vi "Apply Target Pattern.vi"(10 "Mixed Mode Status":T3={"LBCB Target"=[], "MixedModeStates"=enum."Idle", "LBCB Convergence"=[], "LBCB Measurements"=[]}, 11 "Target Pattern":T8) -> (2 "Targets":T1[](array[typedef]))   [LabVIEW 2009]
uses:
  Target Pattern.ctl
  MixedMode/Messages/Target.ctl
  Data Access Objects/Metadata/LBCB Number.ctl
  MixedMode/Messages/Mixed Mode Status.ctl
  MixedMode/Target Data.ctl
  MixedMode/Mixed Mode States.ctl
  MixedMode/Mixed Mode Covergance Status.ctl
  MixedMode/Mixed Mode Cartesian Data.ctl
panel:
  in  "Moments":T1[](array[typedef])=[{"LBCB Number"=enum."LBCB1", "DOF Vectors"=enum."Mx", "Amount"=0.0}, {"LBCB Number"=enum."LBCB1", "DOF Vectors"=enum."My", "Amount"=0.0}, {"LBCB Number"=enum."LBCB1", "DOF Vectors"=enum."Mz", "Amount"=0.0}, {"LBCB Number"=enum."LBCB2", "DOF Vectors"=enum."Mx", "Amount"=0.0}, {"LBCB Number"=enum."LBCB2", "DOF Vectors"=enum."My", "Amount"=0.0}, {"LBCB Number"=enum."LBCB2", "DOF Vectors"=enum."Mz", "Amount"=0.0}]
  in  "Forces":T1[](array[typedef])=[{"LBCB Number"=enum."LBCB1", "DOF Vectors"=enum."Fx", "Amount"=0.0}, {"LBCB Number"=enum."LBCB1", "DOF Vectors"=enum."Fy", "Amount"=0.0}, {"LBCB Number"=enum."LBCB1", "DOF Vectors"=enum."Fz", "Amount"=0.0}, {"LBCB Number"=enum."LBCB2", "DOF Vectors"=enum."Fx", "Amount"=0.0}, {"LBCB Number"=enum."LBCB2", "DOF Vectors"=enum."Fy", "Amount"=0.0}, {"LBCB Number"=enum."LBCB2", "DOF Vectors"=enum."Fz", "Amount"=0.0}]
  in  "Rotations":T1[](array[typedef])=[{"LBCB Number"=enum."LBCB1", "DOF Vectors"=enum."Rx", "Amount"=0.0}, {"LBCB Number"=enum."LBCB1", "DOF Vectors"=enum."Ry", "Amount"=0.0}, {"LBCB Number"=enum."LBCB1", "DOF Vectors"=enum."Rz", "Amount"=0.0}, {"LBCB Number"=enum."LBCB2", "DOF Vectors"=enum."Rx", "Amount"=0.0}, {"LBCB Number"=enum."LBCB2", "DOF Vectors"=enum."Ry", "Amount"=0.0}, {"LBCB Number"=enum."LBCB2", "DOF Vectors"=enum."Rz", "Amount"=0.0}]
  in  "Displacements":T1[](array[typedef])=[{"LBCB Number"=enum."LBCB1", "DOF Vectors"=enum."Dx", "Amount"=0.0}, {"LBCB Number"=enum."LBCB1", "DOF Vectors"=enum."Dy", "Amount"=0.0}, {"LBCB Number"=enum."LBCB1", "DOF Vectors"=enum."Dz", "Amount"=0.0}, {"LBCB Number"=enum."LBCB2", "DOF Vectors"=enum."Dx", "Amount"=0.0}, {"LBCB Number"=enum."LBCB2", "DOF Vectors"=enum."Dy", "Amount"=0.0}, {"LBCB Number"=enum."LBCB2", "DOF Vectors"=enum."Dz", "Amount"=0.0}]
  in  "Reset Zero":T1[](array[typedef])=[{"LBCB Number"=enum."LBCB1", "DOF Vectors"=enum."Dx", "Amount"=0.0}, {"LBCB Number"=enum."LBCB1", "DOF Vectors"=enum."Dy", "Amount"=0.0}, {"LBCB Number"=enum."LBCB1", "DOF Vectors"=enum."Dz", "Amount"=0.0}, {"LBCB Number"=enum."LBCB1", "DOF Vectors"=enum."Rx", "Amount"=0.0}, {"LBCB Number"=enum."LBCB1", "DOF Vectors"=enum."Ry", "Amount"=0.0}, {"LBCB Number"=enum."LBCB1", "DOF Vectors"=enum."Rz", "Amount"=0.0}, {"LBCB Number"=enum."LBCB2", "DOF Vectors"=enum."Dx", "Amount"=0.0}, {"LBCB Number"=enum."LBCB2", "DOF Vectors"=enum."Dy", "Amount"=0.0}, {"LBCB Number"=enum."LBCB2", "DOF Vectors"=enum."Dz", "Amount"=0.0}, {"LBCB Number"=enum."LBCB2", "DOF Vectors"=enum."Rx", "Amount"=0.0}, {"LBCB Number"=enum."LBCB2", "DOF Vectors"=enum."Ry", "Amount"=0.0}, {"LBCB Number"=enum."LBCB2", "DOF Vectors"=enum."Rz", "Amount"=0.0}]
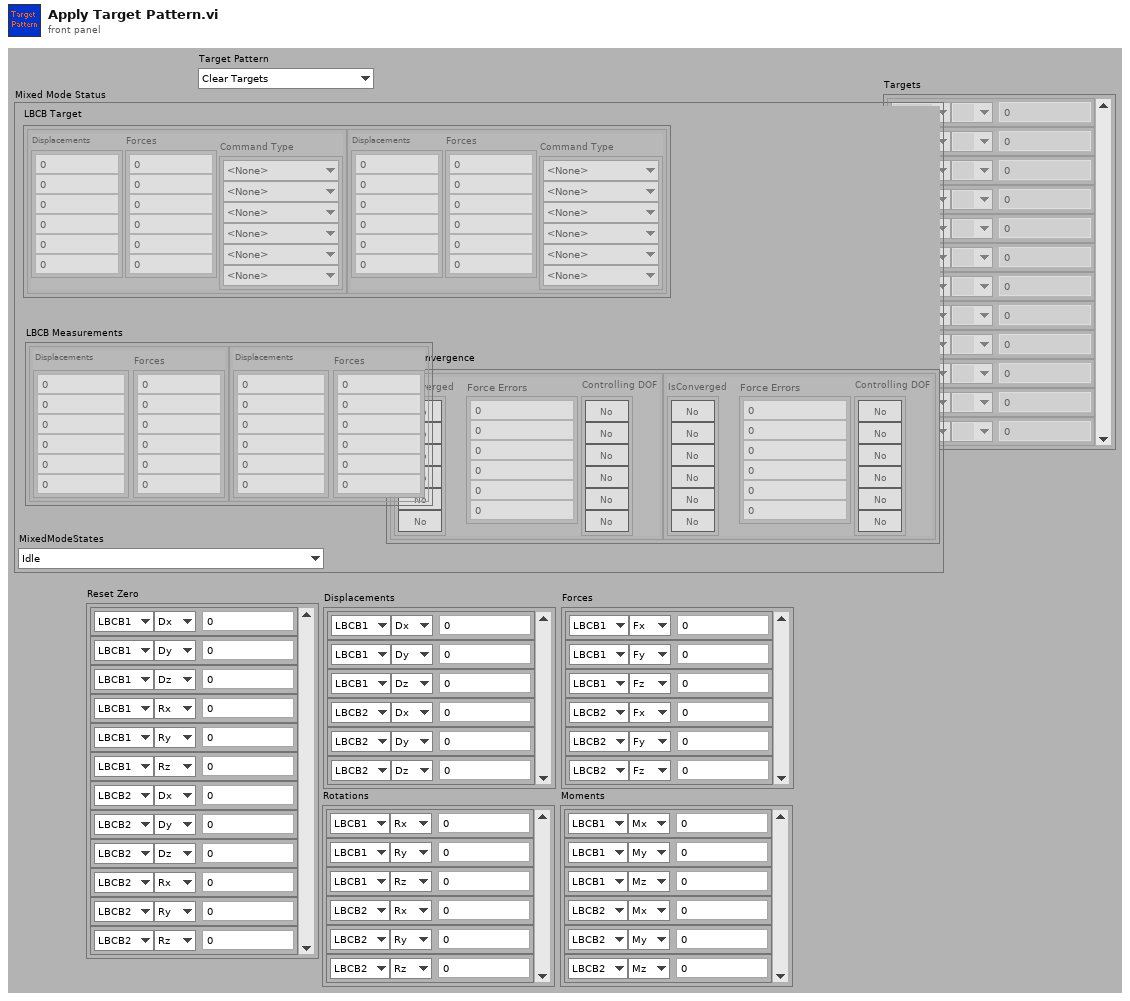
[diagram p1: front panel]
types:
  T1 = typedef "Target.ctl" = cluster{"LBCB Number":T2, "DOF Vectors":enum16{" ", "Dx", "Dy", "Dz", "Rx", "Ry", "Rz", "Fx", "Fy", "Fz", "Mx", "My", "Mz"}, "Amount":dbl}
  T2 = typedef "LBCB Number.ctl" = enum16{"LBCB1", "LBCB2"}
  T3 = typedef "Mixed Mode Status.ctl" = cluster{"LBCB Target":T4[], "MixedModeStates":T5, "LBCB Convergence":T6[], "LBCB Measurements":T7[]}
  T4 = typedef "Target Data.ctl" = cluster{"Displacements":dbl[], "Command Type":enum16{"<None>", "Displacement", "Force"}[], "Forces":dbl[]}
  T5 = typedef "Mixed Mode States.ctl" = enum16{"Init", "Wait For DAQ", "Idle", "Start Initial Position", "Initial Position", "Start Initial Ramp", "Run Initial Ramp", "Start Iterative Stage", "Convergence Check", "Update Stiffness Jacobian", "Update Command", "Start Iterative Ramp", "Run Iterative Ramp", "Start Iterative Stabilize", "Iterative Stabilize", "Start Iterative Holding", "Iterative Holding", "Start Stabilize", "Stabilize", "Start Hold", "Holding", "Done", "Aborting", "Exit", "Nop"}
  T6 = typedef "Mixed Mode Covergance Status.ctl" = cluster{"IsConverged":bool[], "Force Errors":dbl[], "Controlling DOF":bool[]}
  T7 = typedef "Mixed Mode Cartesian Data.ctl" = cluster{"Displacements":dbl[], "Forces":dbl[]}
  T8 = typedef "Target Pattern.ctl" = enum16{"Clear Targets", "Reset Targets to Zero", "Displacements Only", "Rotations Only", "Displacements & Rotations", "Forces Only", "Moments Only", "Forces & Moments"}
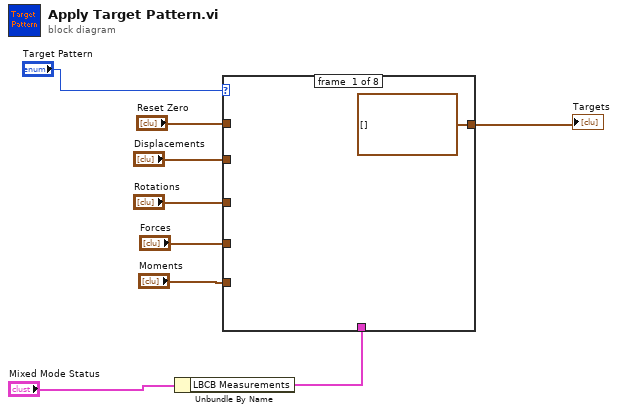
[diagram p0: block diagram]
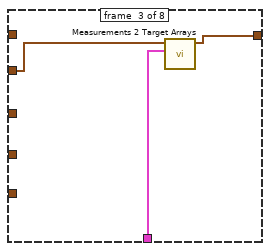
[diagram p3: hidden frame]
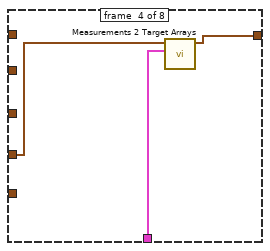
[diagram p4: hidden frame]
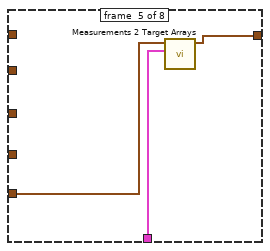
[diagram p5: hidden frame]
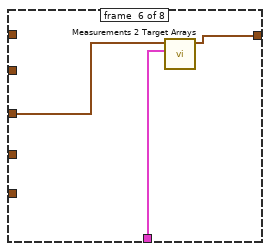
[diagram p6: hidden frame]
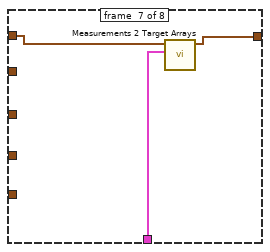
[diagram p7: hidden frame]
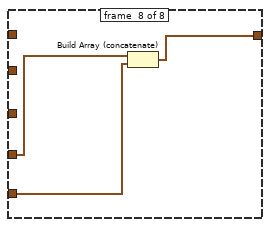
[diagram p8: hidden frame]
diagram:
  n1 = Unbundle By Name("Mixed Mode Status") -> ("LBCB Measurements"=w5:T7[])
  n2 = case shown="\"Forces & Moments\"" "Target Pattern" {
    tunnel: [T1[] [] ("Reset Zero") w11 w12 w16 w19 w22 w25 w27] -> w3
    tunnel: "Reset Zero" -> [_ w11 _ _ _ _ w24 _]
    tunnel: "Displacements" -> [_ _ w14 _ _ _ _ _]
    tunnel: w5 -> [_ _ w13 w17 w20 w23 w26 _]
    tunnel: "Rotations" -> [_ _ _ _ _ w21 _ _]
    tunnel: "Forces" -> [_ _ _ w15 _ _ _ w29]
    tunnel: "Moments" -> [_ _ _ _ w18 _ _ w28]
    frame #0 {
    }
    frame #1 {
    }
    frame #2 {
      n3 = call "Measurements 2 Target Arrays.vi"("LBCB Command Data"=w13, "Target  Inputs"=w14) -> ("Target  Outputs"=w12:T1[])  [unwired: 1 in, 8 out]
    }
    frame #3 {
      n4 = call "Measurements 2 Target Arrays.vi"("LBCB Command Data"=w17, "Target  Inputs"=w15) -> ("Target  Outputs"=w16:T1[])  [unwired: 1 in, 8 out]
    }
    frame #4 {
      n5 = call "Measurements 2 Target Arrays.vi"("LBCB Command Data"=w20, "Target  Inputs"=w18) -> ("Target  Outputs"=w19:T1[])  [unwired: 1 in, 8 out]
    }
    frame #5 {
      n6 = call "Measurements 2 Target Arrays.vi"("LBCB Command Data"=w23, "Target  Inputs"=w21) -> ("Target  Outputs"=w22:T1[])  [unwired: 1 in, 8 out]
    }
    frame #6 {
      n7 = call "Measurements 2 Target Arrays.vi"("LBCB Command Data"=w26, "Target  Inputs"=w24) -> ("Target  Outputs"=w25:T1[])  [unwired: 1 in, 8 out]
    }
    frame #7 {
      n8 = Build Array (concatenate)(w29, w28) -> (w27:T1[])
    }
  }
  "Targets" <- w3
